vi "Host_GUI_Tracking.vi"() -> ()   [LabVIEW 2016]
uses:
  <vilib>/silver_ctls/ArrayMatrixCluster/Real Matrix NI_Silver.ctl
  <vilib>/Analysis/1siggen.llb/Ramp Pattern by Samples.vi
  <vilib>/Analysis/baseanly.llb/Full Cholesky Factorization.vi
  <vilib>/Analysis/baseanly.llb/Full Real Matrix Cholesky Factorization.vi
  <vilib>/Analysis/baseanly.llb/Mean (DBL).vi
  <vilib>/Analysis/7linalg.llb/Real Cholesky Factorization.vi
  <vilib>/Analysis/Matrix/Numeric/Conversions/Array To Matrix - RA2.vi
  <vilib>/Analysis/BLAS.llb/dasum - Absolute Values Sum (DBL).vi
  <vilib>/Analysis/NI_AALBase.lvlib
  <vilib>/gmath/NI_Gmath.lvlib
  <vilib>/Analysis/NI_AALPro.lvlib
  <vilib>/Analysis/NI_AALBLAS.lvlib
  <vilib>/Analysis/Matrix/NI_Matrix.lvlib
  <vilib>/Analysis/Matrix/Datatypes/RealMatrix.ctl
panel:
  out "L4_out":dbl[][](array[numeric])
  out "L3_out":dbl[][](array[numeric])
  out "L2_out":dbl[][](array[numeric])
  out "L1_out":dbl[][](array[numeric])
  out "Zi":dbl[][](array[numeric])
  out "Zp":dbl[][](array[numeric])
  out "Za":dbl[][](array[numeric])
  out "Y":dbl[][](array[numeric])
  out "X":dbl[][](array[numeric])
  out "x_out":dbl[][](array[numeric])
  out "y_out":dbl[][](array[numeric])
  out "z_out":dbl[][](array[numeric])
  out "Tool Rotation":dbl[][](array[numeric])
  out "vacf_out":dbl[][](array[numeric])
  out "time (at via pts)":dbl[][](array[numeric])
  in  "Tab Control":T1(tab)
  out "zi":dbl=5.0 format="%#_3g"
  out "zp_true":dbl=5.0 format="%#_3g"
  out "zp_work":dbl=5.0 format="%#_3g"
  out "za_work":dbl=5.0 format="%#_3g"
  out "za_true":dbl=5.0 format="%#_3g"
  in  "Reflective Index":dbl=1.35 format="%#_13g"
  out "Semi-Axes [mm]":T2
  out "Lens Thickness [mm]":dbl format="%#_3g"
  out "Iris Center [mm]":dbl[](array[numeric]) format="%#_3g"
  in  "Half Span Angle":dbl=60.0
  in  "Radial Attenuation":dbl=0.2 min=0.0 max=1.0 step=0.1
  in  "XY Safety Gap [mm]":dbl=1.5 format="%#_13g"
  out "Avg Iris z_coord [mm]":dbl=-2.0 format="%#_3g"
  in  "Cycle Time [sec]":dbl[](array[numeric])=[60.0, 90.0, 120.0]
  in  "Sampling Rate [Hz]":i32=1000
  out "Za Safety Gap [mm]":dbl[](array[numeric]) format="%#_3g"
  out "Zp Safety Gap [mm]":dbl[](array[numeric]) format="%#_3g"
  in  "Depth Ctrl Array\n(% Thickness)":dbl[](array[numeric])=[20.0, 30.0, 40.0] min=10.0 max=90.0 step=5.0 format="%#_g%%"
  in  "Trajectory Pattern":enum16{"Entry Site", "Centered"}(ring)=enum."Centered"
  in  "No. of Lobes":dbl=10.0
  in  "Radial Offset":dbl=0.2 min=0.0 max=1.0
  in  "Dist Iris2Front [mm]":dbl[](array[numeric])=[0.1, 0.1, 0.1]
  out "No. of Cycles":i32
  out "Total Time [sec]":dbl
  out "Theta1 Waveform Graph":dbl[](graph)
  out "Theta2 Waveform Graph":dbl[](graph)
  out "Theta3 Waveform Graph":dbl[](graph)
  out "Theta4 Waveform Graph":dbl[](graph)
  in  "vac_bnd":dbl[](array[numeric])=[80.0, 100.0]
  in  "z_thld":dbl[](array[numeric])=[0.5, 2.0]
  out "Vacuum Waveform Graph":dbl[](graph)
  out "Ygrid":dbl[](array[numeric])
  out "Xgrid":dbl[](array[numeric])
  in  "OCT z_orgin [mm]":dbl format="%#_13g"
  in  "OCT z_cornea [mm]":dbl format="%#_13g"
  in  "OCT z_post [mm]":dbl format="%#_13g"
  out "Trajectory Length [mm]":dbl[](array[numeric])
  out "Traj Px Waveform Graph":dbl[](graph)
  out "Traj Py Waveform Graph":dbl[](graph)
  out "Traj Pz Waveform Graph":dbl[](graph)
  out "Theta4 Overlaid":dbl[][](graph)
  out "Theta3 Overlaid":dbl[][](graph)
  out "Theta2 Overlaid":dbl[][](graph)
  out "Theta1 Overlaid":dbl[][](graph)
  # "Workspace Parameters"
  # "Top View:"
  # "Cross-Sectioned View:"
  # "No-fly Zone"
  # "Entry Site Pattern"
  # "Centered Pattern"
  # "Z Workspace"
  # "Temporal"
  # "OCT Settings"
  # "XY 2D Grid"
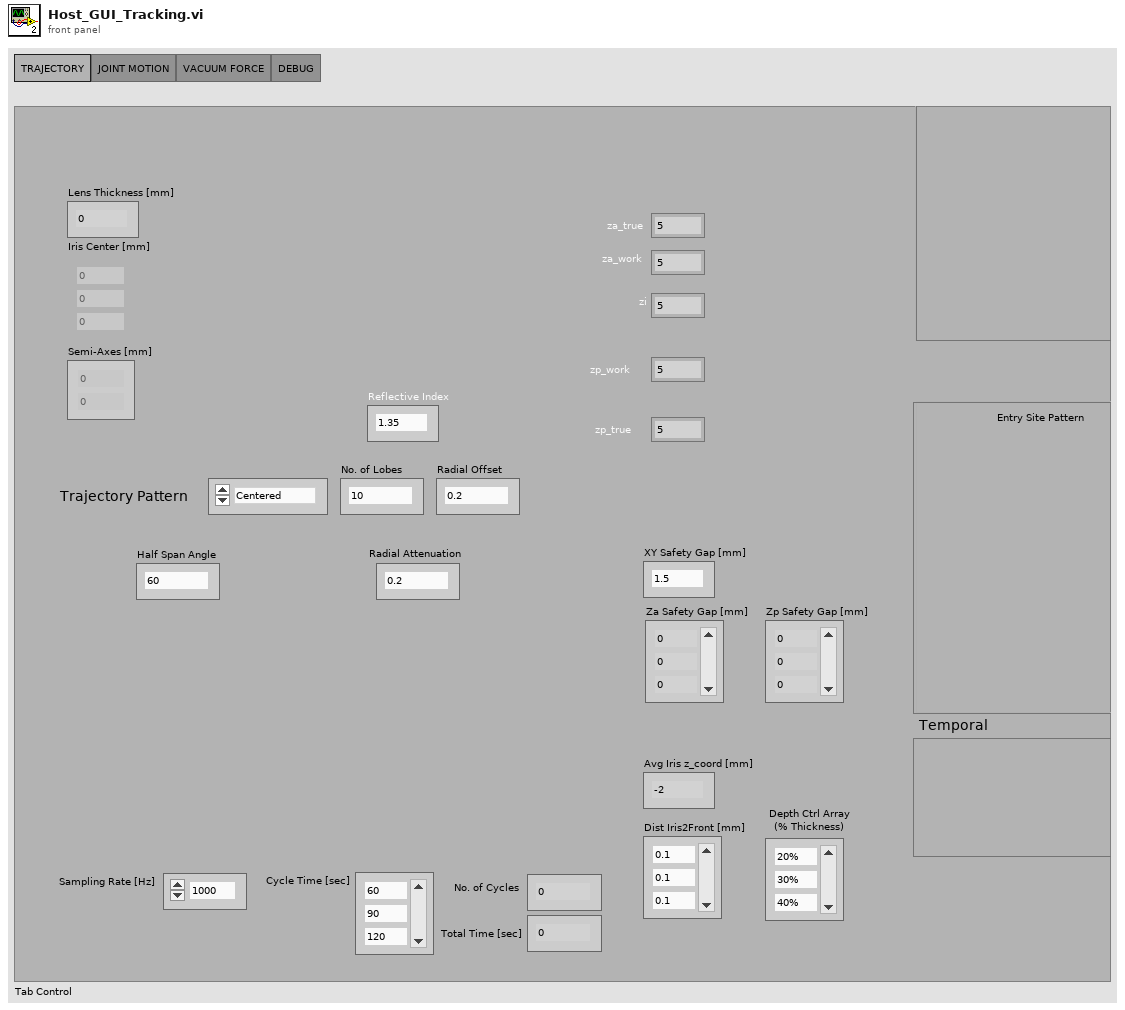
[diagram p1: front panel]
types:
  T1 = enum32{"TRAJECTORY", "JOINT MOTION", "VACUUM FORCE", "DEBUG"}
  T2 = typedef "Real Matrix NI_Silver.ctl" = dbl[][]
  T3 = typedef "NI_Matrix.lvlib/RealMatrix.ctl" = dbl[][]
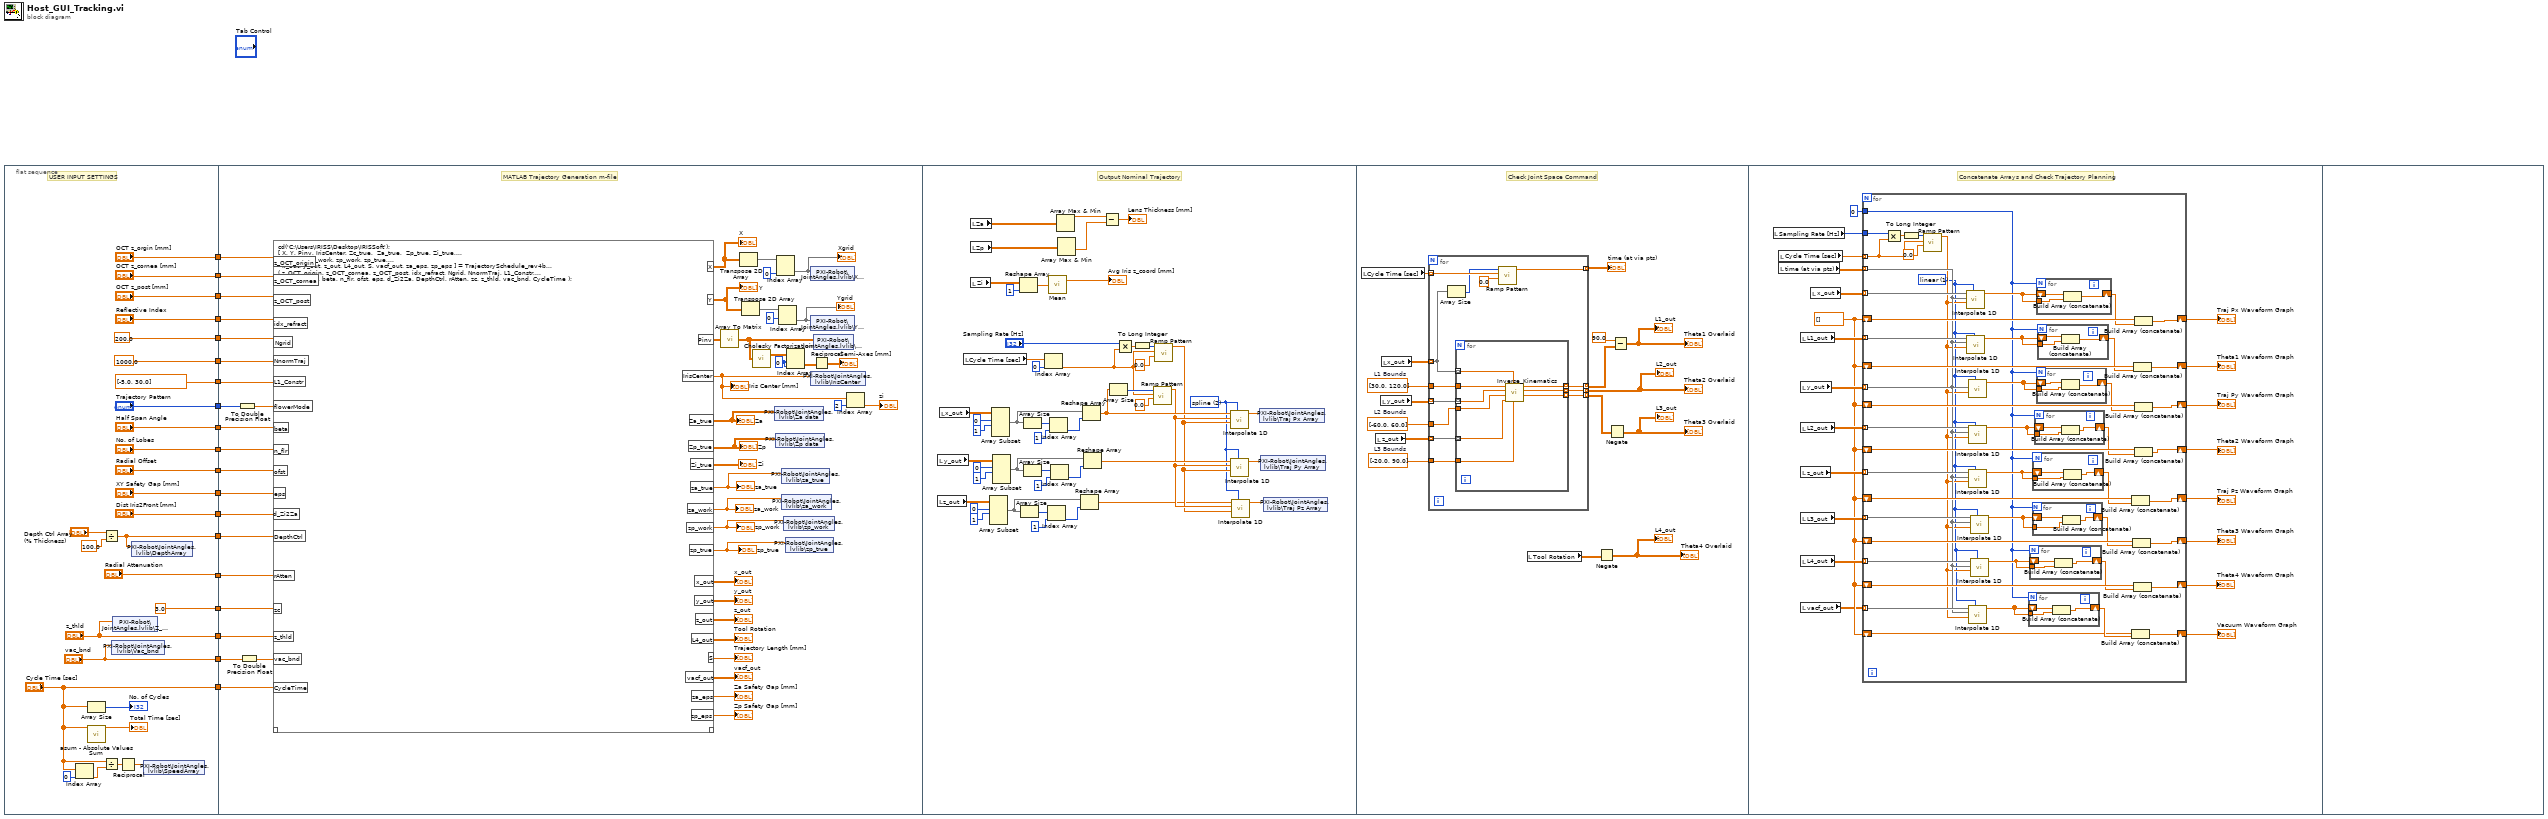
[diagram p0: block diagram]
diagram:
  n1 = flat-sequence {
    tunnel: [200.0 ("Real")] -> w19
    tunnel: ["No. of Lobes"] -> w18
    tunnel: ["Radial Offset"] -> w17
    tunnel: ["XY Safety Gap [mm]"] -> w16
    tunnel: ["Half Span Angle"] -> w15
    tunnel: [1000.0 ("Real")] -> w14
    tunnel: ["z_thld"] -> w13
    tunnel: ["vac_bnd"] -> w12
    tunnel: [3.0 ("zc")] -> w11
    tunnel: ["OCT z_orgin [mm]"] -> w10
    tunnel: ["OCT z_cornea [mm]"] -> w9
    tunnel: ["Reflective Index"] -> w8
    tunnel: ["Trajectory Pattern"] -> w7
    tunnel: ["Dist Iris2Front [mm]"] -> w6
    tunnel: [w22] -> w5
    tunnel: ["Radial Attenuation"] -> w4
    tunnel: ["OCT z_post [mm]"] -> w3
    tunnel: [dbl[] [-5.0, 30.0] ("z_thld")] -> w2
    tunnel: ["Cycle Time [sec]"] -> w1
    tunnel: w19 -> [w94]
    tunnel: w18 -> [w99]
    tunnel: w17 -> [w98]
    tunnel: w16 -> [w97]
    tunnel: w15 -> [w88]
    tunnel: w14 -> [w84]
    tunnel: w13 -> [w83]
    tunnel: w12 -> [w81]
    tunnel: w11 -> [w79]
    tunnel: w10 -> [w77]
    tunnel: w9 -> [w76]
    tunnel: w8 -> [w75]
    tunnel: w7 -> [w74]
    tunnel: w6 -> [w66]
    tunnel: w5 -> [w67]
    tunnel: w4 -> [w72]
    tunnel: w3 -> [w68]
    tunnel: w2 -> [w63]
    tunnel: w1 -> [w61]
    frame #0 {
      # "USER INPUT SETTINGS"
      n2 = Index Array(array="Cycle Time [sec]", index=0) -> (element=w20:dbl)
      n3 = Array Size(array="Cycle Time [sec]") -> (size(s)=→"No. of Cycles":i32)
      n4 = call-poly <vilib>:"asum - Absolute Values Sum.vi"("x"="Cycle Time [sec]") -> ("dasum"=→"Total Time [sec]":dbl)  [unwired: 9 in, 1 out]
      n5 = Divide(x="Depth Ctrl Array\n(% Thickness)", y=100.0) -> (x/y=w22:dbl[])
      n6 = Divide(x="Cycle Time [sec]", y=w20) -> (x/y=w25:dbl[])
      n7 = shared-variable "PXI-Robot\\JointAngles.lvlib\\Vac_bnd"("vac_bnd") -> ()  [unwired: 1 in, 1 out]
      n8 = shared-variable "PXI-Robot\\JointAngles.lvlib\\Z_thld"("z_thld") -> ()  [unwired: 1 in, 1 out]
      n9 = Reciprocal(x=w25) -> (1/x=w24:dbl[])
      n10 = shared-variable "PXI-Robot\\JointAngles.lvlib\\DepthArray"(w22) -> ()  [unwired: 1 in, 1 out]
      n11 = shared-variable "PXI-Robot\\JointAngles.lvlib\\SpeedArray"(w24) -> ()  [unwired: 1 in, 1 out]
    }
    frame #1 {
      w57 = 0 ("index (row)")
      # "Outputs:\n% X: X 2D grid\n% Y: Y 2D grid\n% Pinv: inv(P) for XY ellipse representation\n% IrisCenter: 3-by-1 vector representing the center of iris\n% Zc_true: cornea surface\n% Za_true: anterior surface\n% Zp_true: posterior surface\n% Zi_true: iris plane\n% za_true: center z coordinate of AC\n% za_work: center z coordinate of workspace upper bound\n% zp_work: center z coordinate of workspace lower bound\n% zp_true: center z coordinate of PC\n% x_out: trajectory x position array\n% y_out: trajectory y position array\n% z_out: trajectory z position array\n% L4_out: tool rotation array\n% S: total arc length\n% vacf_out: vacuum scheduling array\n% za_eps: anterior safety gap\n% zp_eps: posterior safety gap\n\nInputs:\n% z_OCT_origin: where OCT performs 20-pt algorithm for coord. transformation\n% z_OCT_cornea: where OCT takes a snap shot for cornea\n% z_OCT_post: where OCT takes a snap shot for posterior capsule\n% idx_refract: refractive index\n% Ngrid: no. of XY grid points\n% Ntraj: no. of points used for trajectory generation\n% L1_Constr: constraint on L1 angles\n% flowerMode: flower pattern selection\n% beta: half angle range in deg on z=zi plane\n% n_flr: no. of lobes (even)\n% ofst: relative offset of flower pattern from starting point\n% eps:  safety gap thickness in XY in mm\n% d_Zi2Za: distance to anterior capsule\n% DepthCtrl: depth control in terms of thickness for each stage\n% zc: axis of aspiration points towards (0,~,zc)\n% z_thld: threshold z distances used to define extreme values of vacuum force\n% vac_bnd: extreme values of vacuum force\n% CycleTime: time elapsed per cycle"
      # "MATLAB Trajectory Generation m-file"
      n12 = To Double Precision Float(number=w74) -> (double precision float=w73:dbl)
      n13 = To Double Precision Float(number=w81) -> (double precision float=w80:dbl[])
      n14 = script code="cd('C:\\Users\\IRISS\\Desktop\\IRISSoft');\n[ X, Y, Pinv, IrisCenter, Zc_true,  Za_true,  Zp_true, Zi_true,...\n  za_true, za_work, zp_work, zp_true,...\n  x_out, y_out, z_out, L4_out, S, vacf_out, za_eps, zp_eps ] = TrajectorySchedule_rev4b...\n( z_OCT_origin, z_OCT_cornea, z_OCT_post, idx_refract, Ngrid, NnormTraj, L1_Constr,...\n  flowerMode, beta, n_flr, ofst, eps, d_Zi2Za, DepthCtrl, rAtten, zc, z_thld, vac_bnd, CycleTime );"("Ngrid"=w94, "n_flr"=w99, "ofst"=w98, "eps"=w97, "beta"=w88, "zc"=w79, "NnormTraj"=w84, "z_thld"=w83, "vac_bnd"=w80, "idx_refract"=w75, "z_OCT_cornea"=w76, "z_OCT_origin"=w77, "flowerMode"=w73, "d_Zi2Za"=w66, "DepthCtrl"=w67, "rAtten"=w72, "z_OCT_post"=w68, "L1_Constr"=w63, "CycleTime"=w61) -> ("x_out"=→"x_out":dbl[][], "y_out"=→"y_out":dbl[][], "z_out"=→"z_out":dbl[][], "S"=→"Trajectory Length [mm]":dbl[], "X"=w86:dbl[][], "Y"=w90:dbl[][], "Zp_true"=w78:dbl[][], "Za_true"=w85:dbl[][], "L4_out"=→"Tool Rotation":dbl[][], "vacf_out"=→"vacf_out":dbl[][], "Pinv"=w60:dbl[][], "IrisCenter"=w47:dbl[], "Zi_true"=→"Zi":dbl[][], "za_eps"=→"Za Safety Gap [mm]":dbl[], "zp_eps"=→"Zp Safety Gap [mm]":dbl[], "za_true"=w51:dbl, "za_work"=w50:dbl, "zp_work"=w49:dbl, "zp_true"=w48:dbl)  [unwired: 1 in, 1 out]
      "X" <- w86
      "Y" <- w90
      "Zp" <- w78
      "Za" <- w85
      "Iris Center [mm]" <- w47
      "za_true" <- w51
      "za_work" <- w50
      "zp_work" <- w49
      "zp_true" <- w48
      n15 = call-poly <vilib>:"Array To Matrix.vi"("Real 2D Array"=w60) -> ("Real Matrix"=w59:T3)
      n16 = Transpose 2D Array(2D array=w86) -> (transposed array=w93:dbl[][])
      n17 = Transpose 2D Array(2D array=w90) -> (transposed array=w91:dbl[][])
      n18 = call-poly <vilib>:"Cholesky Factorization.vi"("A"=w59) -> ("Cholesky"=w58:T3)  [unwired: 1 out]
      n19 = shared-variable "PXI-Robot\\JointAngles.lvlib\\Za data"(w85) -> ()  [unwired: 1 in, 1 out]
      n20 = shared-variable "PXI-Robot\\JointAngles.lvlib\\Zp data"(w78) -> ()  [unwired: 1 in, 1 out]
      n21 = Index Array(array=w93, index (col)=0 ("disabled index (col)")) -> (element=w70:dbl[])  [unwired: 1 in]
      "Xgrid" <- w70
      n22 = Index Array(array=w91, index (row)=0 ("disabled index (col)")) -> (element=w69:dbl[])  [unwired: 1 in]
      "Ygrid" <- w69
      n23 = shared-variable "PXI-Robot\\JointAngles.lvlib\\za_work"(w50) -> ()  [unwired: 1 in, 1 out]
      n24 = shared-variable "PXI-Robot\\JointAngles.lvlib\\za_true"(w51) -> ()  [unwired: 1 in, 1 out]
      n25 = shared-variable "PXI-Robot\\JointAngles.lvlib\\zp_work"(w49) -> ()  [unwired: 1 in, 1 out]
      n26 = shared-variable "PXI-Robot\\JointAngles.lvlib\\zp_true"(w48) -> ()  [unwired: 1 in, 1 out]
      n27 = Index Array(array=w58, index (row)=w57, index (col)=w57) -> (element=w56:T3)
      n28 = shared-variable "PXI-Robot\\JointAngles.lvlib\\IrisCenter"(w47) -> ()  [unwired: 1 in, 1 out]
      n29 = shared-variable "PXI-Robot\\JointAngles.lvlib\\X grid"(w70) -> ()  [unwired: 1 in, 1 out]
      n30 = shared-variable "PXI-Robot\\JointAngles.lvlib\\Y grid"(w69) -> ()  [unwired: 1 in, 1 out]
      n31 = Reciprocal(x=w56) -> (1/x=→"Semi-Axes [mm]":T3)
      n32 = shared-variable "PXI-Robot\\JointAngles.lvlib\\Pinv"(w59) -> ()  [unwired: 1 in, 1 out]
      n33 = Index Array(array=w47, index=2) -> (element=→"zi":dbl)
    }
    frame #2 {
      w104 = 2 items=["nearest", "linear", "spline", "cubic Hermite", "Lagrange"] ("method")
      # "Output Nominal Trajectory"
      n34 = local read "z_out"() -> (w122:dbl[][])
      n35 = local read "y_out"() -> (w132:dbl[][])
      n36 = local read "x_out"() -> (w133:dbl[][])
      n37 = local read "Cycle Time [sec]"() -> (w118:dbl[])
      n38 = local read "Za"() -> (w147:dbl[][])
      n39 = local read "Zp"() -> (w146:dbl[][])
      n40 = local read "Zi"() -> (w142:dbl[][])
      n41 = Array Subset(array=w122, index (row)=0 ("index"), length (row)=1 ("length")) -> (w100:dbl[][])  [unwired: 2 in]
      n42 = Array Subset(array=w133, index (row)=0 ("index"), length (row)=1 ("length")) -> (w136:dbl[][])  [unwired: 2 in]
      n43 = Array Subset(array=w132, index (row)=0 ("index"), length (row)=1 ("length")) -> (w129:dbl[][])  [unwired: 2 in]
      n44 = Reshape Array(w142, 1 ("dimension size")) -> (w140:dbl[])
      n45 = Array Size(array=w100) -> (size(s)=w124:i32[])
      n46 = Array Size(array=w136) -> (size(s)=w135:i32[])
      n47 = Array Size(array=w129) -> (size(s)=w130:i32[])
      n48 = Index Array(array=w118, index=0) -> (element=w109:dbl)
      n49 = Index Array(array=w124, index=1) -> (element=w123:i32)
      n50 = call-poly <vilib>:"Mean.vi"("X"=w140) -> ("mean"=→"Avg Iris z_coord [mm]":dbl)  [unwired: 1 out]
      n51 = Index Array(array=w135, index=1) -> (element=w134:i32)
      n52 = Index Array(array=w130, index=1) -> (element=w131:i32)
      n53 = Array Max & Min(array=w147) -> (max value=w145:dbl)  [unwired: 3 out]
      n54 = Array Max & Min(array=w146) -> (min value=w144:dbl)  [unwired: 3 out]
      n55 = Reshape Array(w100, w123) -> (w101:dbl[])
      n56 = Reshape Array(w136, w134) -> (w110:dbl[])
      n57 = Reshape Array(w129, w131) -> (w108:dbl[])
      n58 = Subtract(x=w145, y=w144) -> (x-y=→"Lens Thickness [mm]":dbl)
      n59 = Array Size(array=w110) -> (size(s)=w111:i32)
      n60 = Multiply(x="Sampling Rate [Hz]", y=w109) -> (x*y=w114:dbl)
      n61 = To Long Integer(number=w114) -> (32bit integer=w115:i32)
      n62 = call-poly <vilib>:"Ramp Pattern.vi"("start"=0.0, "end"=w109, "samples"=w111) -> ("Ramp Pattern"=w107:dbl[])  [unwired: 7 in, 1 out]
      n63 = call-poly <vilib>:"Ramp Pattern.vi"("start"=0.0, "end"=w109, "samples"=w115) -> ("Ramp Pattern"=w106:dbl[])  [unwired: 7 in, 1 out]
      n64 = call <vilib>:"Interpolate 1D.vi"("method"=w104, "xi"=w106, "X"=w107, "Y"=w110) -> ("yi"=w103:dbl[])  [unwired: 5 in, 2 out]
      n65 = call <vilib>:"Interpolate 1D.vi"("method"=w104, "xi"=w106, "X"=w107, "Y"=w108) -> ("yi"=w105:dbl[])  [unwired: 5 in, 2 out]
      n66 = call <vilib>:"Interpolate 1D.vi"("method"=w104, "xi"=w106, "X"=w107, "Y"=w101) -> ("yi"=w102:dbl[])  [unwired: 5 in, 2 out]
      n67 = shared-variable "PXI-Robot\\JointAngles.lvlib\\Traj Px Array"(w103) -> ()  [unwired: 1 in, 1 out]
      n68 = shared-variable "PXI-Robot\\JointAngles.lvlib\\Traj Py Array"(w105) -> ()  [unwired: 1 in, 1 out]
      n69 = shared-variable "PXI-Robot\\JointAngles.lvlib\\Traj Pz Array"(w102) -> ()  [unwired: 1 in, 1 out]
    }
    frame #3 {
      w161 = dbl[] [-20.0, 90.0]  # L3 Bounds
      w162 = dbl[] [-60.0, 60.0]  # L2 Bounds
      w163 = dbl[] [30.0, 120.0]  # L1 Bounds
      # "Check Joint Space Command"
      n70 = local read "Cycle Time [sec]"() -> (w148:dbl[])
      n71 = local read "z_out"() -> (w158:dbl[][])
      n72 = local read "y_out"() -> (w159:dbl[][])
      n73 = local read "x_out"() -> (w160:dbl[][])
      n74 = for {
        tunnel: w148 -> [w175] mode=indexing
        tunnel: w163 -> [w174]
        tunnel: w162 -> [w173]
        tunnel: w161 -> [w172]
        tunnel: w160 -> [w166] mode=indexing
        tunnel: w159 -> [w171] mode=indexing
        tunnel: w158 -> [w170] mode=indexing
        tunnel: [w169] -> w155 mode=indexing
        tunnel: [w168] -> w154 mode=indexing
        tunnel: [w167] -> w152 mode=indexing
        tunnel: [w164] -> w157 mode=indexing
        n75 = Array Size(array=w166) -> (size(s)=w165:i32)
        n76 = for {
          tunnel: w174 -> [w185]
          tunnel: w173 -> [w184]
          tunnel: w172 -> [w183]
          tunnel: w166 -> [w182] mode=indexing
          tunnel: w171 -> [w181] mode=indexing
          tunnel: w170 -> [w180] mode=indexing
          tunnel: [w179] -> w169 mode=indexing
          tunnel: [w178] -> w168 mode=indexing
          tunnel: [w177] -> w167 mode=indexing
          n77 = call "Inverse_Kinematics.vi"("B3"=w183, "px"=w182, "pz"=w180, "B2"=w184, "py"=w181, "B1"=w185) -> ("theta 3"=w177:dbl, "theta 2"=w178:dbl, "theta 1"=w179:dbl)  [unwired: 1 out]
        }
        n78 = call-poly <vilib>:"Ramp Pattern.vi"("start"=0.0, "end"=w175, "samples"=w165) -> ("Ramp Pattern"=w164:dbl[])  [unwired: 7 in, 1 out]
      }
      "L2_out" <- w154
      "time (at via pts)" <- w157
      "Theta2 Overlaid" <- w154
      n79 = local read "Tool Rotation"() -> (w153:dbl[][])
      n80 = Negate(x=w153) -> (-x=→"Theta4 Overlaid" →"L4_out":dbl[][])
      n81 = Negate(x=w152) -> (-x=→"L3_out" →"Theta3 Overlaid":dbl[][])
      n82 = Subtract(x=90.0, y=w155) -> (x-y=→"L1_out" →"Theta1 Overlaid":dbl[][])
    }
    frame #4 {
      w187 = dbl[] []
      # "Concatenate Arrays and Check Trajectory Planning"
      n83 = local read "Sampling Rate [Hz]"() -> (w189:i32)
      n84 = local read "Cycle Time [sec]"() -> (w204:dbl[])
      n85 = local read "time (at via pts)"() -> (w206:dbl[][])
      n86 = local read "L1_out"() -> (w203:dbl[][])
      n87 = local read "y_out"() -> (w202:dbl[][])
      n88 = local read "L2_out"() -> (w201:dbl[][])
      n89 = local read "z_out"() -> (w200:dbl[][])
      n90 = local read "L3_out"() -> (w199:dbl[][])
      n91 = local read "L4_out"() -> (w198:dbl[][])
      n92 = local read "vacf_out"() -> (w186:dbl[][])
      n93 = local read "x_out"() -> (w205:dbl[][])
      n94 = for {
        tunnel: w206 -> [w211] mode=indexing
        tunnel: w205 -> [w255] mode=indexing
        tunnel: w204 -> [w247] mode=indexing
        tunnel: w189 -> [w254]
        tunnel: w203 -> [w252] mode=indexing
        tunnel: w202 -> [w251] mode=indexing
        tunnel: w201 -> [w250] mode=indexing
        tunnel: w200 -> [w249] mode=indexing
        tunnel: w199 -> [w248] mode=indexing
        tunnel: w198 -> [w246] mode=indexing
        shift-right: [w235] -> w197
        shift-left: w187 -> [w236]
        shift-right: [w233] -> w196
        shift-left: w187 -> [w234]
        shift-right: [w231] -> w195
        shift-left: w187 -> [w232]
        shift-right: [w229] -> w194
        shift-left: w187 -> [w230]
        shift-right: [w227] -> w193
        shift-left: w187 -> [w228]
        shift-right: [w226] -> w192
        shift-left: w187 -> [w225]
        shift-right: [w224] -> w191
        shift-left: w187 -> [w223]
        tunnel: 0 ("No. of Cycles") -> [w207]
        shift-right: [w213] -> w188
        shift-left: w187 -> [w208]
        tunnel: w186 -> [w212] mode=indexing
        w209 = 1 items=["nearest", "linear", "spline", "cubic Hermite", "Lagrange"] ("method")
        n95 = Multiply(x=w254, y=w247) -> (x*y=w245:dbl)
        n96 = To Long Integer(number=w245) -> (32bit integer=w244:i32)
        n97 = call-poly <vilib>:"Ramp Pattern.vi"("start"=0.0, "end"=w247, "samples"=w244) -> ("Ramp Pattern"=w210:dbl[])  [unwired: 7 in, 1 out]
        n98 = call <vilib>:"Interpolate 1D.vi"("method"=w209, "xi"=w210, "X"=w211, "Y"=w255) -> ("yi"=w243:dbl[])  [unwired: 5 in, 2 out]
        n99 = call <vilib>:"Interpolate 1D.vi"("method"=w209, "xi"=w210, "X"=w211, "Y"=w252) -> ("yi"=w242:dbl[])  [unwired: 5 in, 2 out]
        n100 = call <vilib>:"Interpolate 1D.vi"("method"=w209, "xi"=w210, "X"=w211, "Y"=w251) -> ("yi"=w241:dbl[])  [unwired: 5 in, 2 out]
        n101 = call <vilib>:"Interpolate 1D.vi"("method"=w209, "xi"=w210, "X"=w211, "Y"=w250) -> ("yi"=w240:dbl[])  [unwired: 5 in, 2 out]
        n102 = call <vilib>:"Interpolate 1D.vi"("method"=w209, "xi"=w210, "X"=w211, "Y"=w249) -> ("yi"=w239:dbl[])  [unwired: 5 in, 2 out]
        n103 = call <vilib>:"Interpolate 1D.vi"("method"=w209, "xi"=w210, "X"=w211, "Y"=w212) -> ("yi"=w214:dbl[])  [unwired: 5 in, 2 out]
        n104 = call <vilib>:"Interpolate 1D.vi"("method"=w209, "xi"=w210, "X"=w211, "Y"=w248) -> ("yi"=w238:dbl[])  [unwired: 5 in, 2 out]
        n105 = call <vilib>:"Interpolate 1D.vi"("method"=w209, "xi"=w210, "X"=w211, "Y"=w246) -> ("yi"=w237:dbl[])  [unwired: 5 in, 2 out]
        n106 = for {
          N: w207 -> [_]
          tunnel: w214 -> [w257]
          shift-right: [w256] -> w215
          shift-left: w214 -> [w258]
          n107 = Build Array (concatenate)(w258, w257) -> (w256:dbl[])
        }
        n108 = for {
          N: w207 -> [_]
          tunnel: w237 -> [w260]
          shift-right: [w259] -> w217
          shift-left: w237 -> [w261]
          n109 = Build Array (concatenate)(w261, w260) -> (w259:dbl[])
        }
        n110 = for {
          N: w207 -> [_]
          shift-right: [w262] -> w218
          shift-left: w238 -> [w264]
          tunnel: w238 -> [w263]
          n111 = Build Array (concatenate)(w264, w263) -> (w262:dbl[])
        }
        n112 = for {
          N: w207 -> [_]
          shift-right: [w265] -> w219
          shift-left: w239 -> [w267]
          tunnel: w239 -> [w266]
          n113 = Build Array (concatenate)(w267, w266) -> (w265:dbl[])
        }
        n114 = for {
          N: w207 -> [_]
          shift-right: [w268] -> w220
          shift-left: w240 -> [w270]
          tunnel: w240 -> [w269]
          n115 = Build Array (concatenate)(w270, w269) -> (w268:dbl[])
        }
        n116 = for {
          N: w207 -> [_]
          shift-right: [w271] -> w221
          shift-left: w241 -> [w273]
          tunnel: w241 -> [w272]
          n117 = Build Array (concatenate)(w273, w272) -> (w271:dbl[])
        }
        n118 = for {
          N: w207 -> [_]
          shift-right: [w279] -> w216
          shift-left: w243 -> [w278]
          tunnel: w243 -> [w277]
          n119 = Build Array (concatenate)(w278, w277) -> (w279:dbl[])
        }
        n120 = for {
          N: w207 -> [_]
          shift-right: [w274] -> w222
          shift-left: w242 -> [w276]
          tunnel: w242 -> [w275]
          n121 = Build Array (concatenate)(w276, w275) -> (w274:dbl[])
        }
        n122 = Build Array (concatenate)(w228, w219) -> (w227:dbl[])
        n123 = Build Array (concatenate)(w208, w215) -> (w213:dbl[])
        n124 = Build Array (concatenate)(w225, w218) -> (w226:dbl[])
        n125 = Build Array (concatenate)(w223, w217) -> (w224:dbl[])
        n126 = Build Array (concatenate)(w234, w222) -> (w233:dbl[])
        n127 = Build Array (concatenate)(w236, w216) -> (w235:dbl[])
        n128 = Build Array (concatenate)(w232, w221) -> (w231:dbl[])
        n129 = Build Array (concatenate)(w230, w220) -> (w229:dbl[])
      }
      "Theta1 Waveform Graph" <- w196
      "Traj Px Waveform Graph" <- w197
      "Theta2 Waveform Graph" <- w194
      "Theta4 Waveform Graph" <- w191
      "Theta3 Waveform Graph" <- w192
      "Traj Py Waveform Graph" <- w195
      "Traj Pz Waveform Graph" <- w193
      "Vacuum Waveform Graph" <- w188
    }
    frame #5 {
    }
  }
